vi "Dashboard Main.vi"() -> ()   [LabVIEW 2020]
uses:
  <vilib>/Utility/miscctls.llb/LVRowAndColumnTypeDef.ctl
  <vilib>/event_ctls.llb/eventvkey.ctl
  <vilib>/Rock Robotics/Network Tables/NT Read Numeric Array.vi
  AUtonomo/Robot Global Data.vi
  <vilib>/Rock Robotics/WPI/Dashboard/WPI_DashboardLogging Global.vi
panel:
  in  "Camera Settings Right":T1={"Frame Rate"=30, "Compression"=30, "Size"=1, "DB Camera Config"=FALSE} {"Frame Rate" scale=1.0..30.0; "Compression" scale=100.0..-1.0; "Size" items=["640x480", "320x240", "160x120"]}
  in  "Camera Name Right":string(combo)="No Camera Selection"
  out "Camera Perf":string
  in  "Camera Settings":T1={"Frame Rate"=30, "Compression"=30, "Size"=1, "DB Camera Config"=FALSE} {"Frame Rate" scale=1.0..30.0; "Compression" scale=100.0..-1.0; "Size" items=["640x480", "320x240", "160x120"]}
  in  "TCP":refnum<k5>
  in  "Rec Mode":enum32{"Stop", "Record", "Playback"}(radio)
  out "Robot IP":string
  out "Image Message":string="Timeout in Camera Communications"
  in  "Dashboard Tab":T2(tab)
  in  "Select Auto":string(combo)="Select Autonomous ..."
  out "NT Connection":bool
  out "MotorChart R":cluster{"Numeric":dbl, "Numeric":dbl}(graph)
  out "MotorChart L":cluster{"Numeric":dbl, "Numeric":dbl}(graph)
  out "MotorSliders R":cluster{"MotorSlide1":dbl, "MotorSlide2":dbl} {"MotorSlide2" scale=-1.0..1.0 scale format="%#_2e"; "MotorSlide1" scale=-1.0..1.0 scale format="%#_2e"}
  out "MotorSliders L":cluster{"MotorSlide1":dbl, "MotorSlide2":dbl} {"MotorSlide2" scale=-1.0..1.0 scale format="%#_2e"; "MotorSlide1" scale=-1.0..1.0 scale format="%#_2e"}
  out "Gyro":dbl(knob) scale=0.0..360.0
  out "JS1 Z":dbl(slide) scale=-1.0..1.0 scale format="%#_2e"
  out "JS1 Graph":cluster{"X":dbl, "Y":dbl}[](graph)
  out "JS1 Buttons":T3
  out "JS2 Z":dbl(slide) scale=-1.0..1.0 scale format="%#_2e"
  out "JS2 Graph":cluster{"X":dbl, "Y":dbl}[](graph)
  out "JS2 Buttons":T3
  out "Mode":T4(ring)=enum."Auto Disabled"
  out "Right Camera Perf":cluster{"Bandwidth (Mbps)":dbl, "FPS":dbl}
  out "Camera Image Right":T5(plugin-control)
  in  "DB/String 9":string
  in  "DB/String 8":string
  in  "DB/String 7":string
  in  "DB/String 6":string
  in  "DB/String 5":string
  in  "DB/String 4":string
  in  "DB/String 3":string
  in  "DB/String 2":string
  in  "DB/String 1":string
  in  "DB/String 0":string
  in  "DB/Slider 0":dbl(slide) scale=0.0..5.0
  in  "DB/Slider 1":dbl(slide) scale=0.0..5.0
  in  "DB/Slider 2":dbl(slide) scale=0.0..5.0
  in  "DB/Slider 3":dbl(slide) scale=0.0..5.0
  out "DB/LED 3":bool
  out "DB/LED 2":bool
  out "DB/LED 1":bool
  out "DB/LED 0":bool
  in  "DB/Button 3":bool
  in  "DB/Button 2":bool
  in  "DB/Button 1":bool
  in  "DB/Button 0":bool caption="New Name"
  in  "Test Slider":dbl(slide) scale=0.0..100.0 scale format="%#_3g"
  in  "On/Off":bool caption="Solenoid"
  in  "Test Name":u16(ring) items=["Select the test to run..."]
  in  "Test Tree":string(tree)
  in  "Motor":cluster{"Value":dbl, "Enable":bool} {"Value" scale=-1.0..1.0 scale format="%#_3g"}
  out "Progress":T6 {"Test Progress" scale=0.0..100.0}
  in  "Rev/Fwd":cluster{"Forward":bool, "Reverse":bool}
  in  "Test Ring":u16(ring) items=["Monochrome", "Color"]
  out "Cmd Status":string
  in  "Execute Command":bool
  in  "Command Params":string[][](table)
  in  "Command Selection":i32(listbox)
  in  "CheckList":i32(listbox)
  out "Tree":string(tree)
  out "Camera Image":T5(plugin-control)
  out "Background":bool
  in  "Camera Name":string(combo)="No Camera Selection"
  # "HW"
  # "HW"
  # "Joysticks"
  # "Drive Motors"
  # "Front"
  # "Right"
  # "Left"
  # "Back"
  # "This tab is a great place for autonomous settings and robot-specific values.\nPlace controls and indicators inside this tab and match name to\nDashboard Variables on robot. You can also delete this comment."
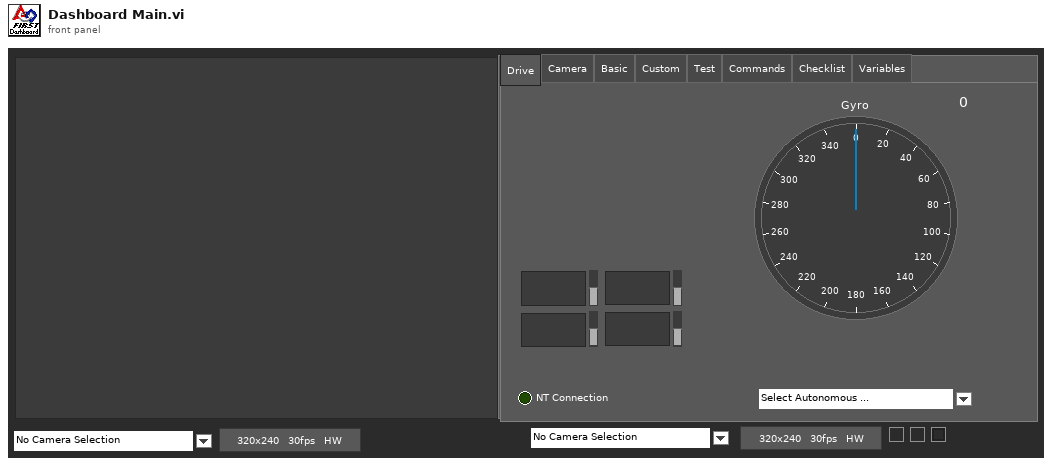
[diagram p1: front panel]
types:
  T1 = cluster{"Frame Rate":i32, "Compression":i32, "Size":u16, "DB Camera Config":bool}
  T2 = enum32{"Drive", "Camera", "Basic", "Custom", "Test", "Commands", "Checklist", "Variables"}
  T3 = cluster{bool, bool, bool, bool, bool, bool, bool, bool, bool, bool, bool, bool}
  T4 = enum8{"Tele-Op Disabled", "Tele-Op Enabled", "Auto Disabled", "Auto Enabled", "Test Disabled", "Test Enabled", "Disconnected", "No Code", "E-Stop"}
  T5 = typedef "IMAQ Image.ctl" = refnum<image>
  T6 = cluster{"Test Progress":u8, "Test Progress Text":string}
  T7 = cluster{"Save Path":path, "Interval (s)":dbl, "Keep":i32}
  T8 = typedef "Image Type" = u32
  T9 = cluster{"IDs":cluster{"RPC field ID":u16, "Unique ID":u16}, "String":string}
  T10 = cluster{"Error Strings":string, "Disable Counts":cluster{u16, u16}, "Rail Faults":cluster{u16, u16, u16}, "Robot IP":string, "DB Mode":u8, "Event Info":cluster{"Name":string, "Type":u8, "Number":u16, "Replay":u8}}
  T11 = cluster{"Storage":cluster{"Disk Free":u64, "RAM Block":u32, "RAM free":u32}, "CPU Utilization":cluster{"CPU % ISR":sgl, "CPU % Time Crit":sgl, "CPU % Timed Str":sgl, "CPU % High":sgl, "CPU % Above":sgl, "CPU % Normal":sgl, "CPU % Low":sgl}, "CAN":cluster{"% Bus Utilization":sgl, "Bus Off Cnt":u32, "TX_FIFO Full Cnt":u32, "Receive Error Cnt":u8, "Transmit Error Cnt":u8}, "HID":cluster{"HID Outputs":u32, "Rumble Low":u16, "Rumble High":u16}[]}
  T12 = cluster{"Status bits":cluster{"Test Mode":bool, "Autonomous":bool, "Enabled":bool, "Code Start":bool, "Brownout":bool, "Reserved 2":bool, "Reserved 3":bool, "E-Stop":bool}, "Code Trace":cluster{"Disabled":bool, "TeleOp":bool, "Auto":bool, "Test":bool}, "Controller Type":enum16{"unknown", "cRIO", "roboRio"}, "Code?":enum16{"unknown", "noCode", "code"}, "Battery V":dbl}
  T13 = cluster{"Control Bits":cluster{"TestMode":bool, "Autonomous":bool, "Enabled":bool, "FMS Present":bool, bool, bool, bool, "E-Stop":bool}, "Team Station ":u8, "Countdown":sgl, "Joystick Values":cluster{"Axes":dbl[], "Buttons":bool[], "POVs":i16[]}[]}
  T14 = cluster{"Axes":dbl[], "Buttons":bool[], "POVs":i16[]}[]
  T15 = cluster{"Axes":dbl[], "Buttons":bool[], "POVs":i16[]}
  T16 = cluster{"Buttons[0]":bool, "Buttons[1]":bool, "Buttons[2]":bool, "Buttons[3]":bool, "Buttons[4]":bool, "Buttons[5]":bool, "Buttons[6]":bool, "Buttons[7]":bool, "Buttons[8]":bool, "Buttons[9]":bool, "Buttons[10]":bool, "Buttons[11]":bool}
  T17 = cluster{"Camera Image":refnum<vi>, "Dashboard Tab":refnum<vi>, "Background":refnum<vi>, "Rec Mode":refnum<vi>, "Test Slider":refnum<vi>, "On/Off ":refnum<vi>, "Test Ring":refnum<vi>, "Rev/Fwd":refnum<vi>, "Test Name":refnum<vi>, "Motor":refnum<vi>, "Progress":refnum<vi>, "CheckList":refnum<vi>, "Tree":refnum<vi>, "Test Tree":refnum<vi>, "Command Params":refnum<vi>, "Command Selection":refnum<vi>, "Execute Command":refnum<vi>, "Cmd Status":refnum<vi>, "Camera Settings":refnum<vi>, "Camera Name":refnum<vi>, "Camera Perf":refnum<vi>, "Camera Settings Right":refnum<vi>, "Camera Name Right":refnum<vi>, "Camera Image Right":refnum<vi>}
  T18 = cluster{"Global Rectangle":i32[], "Contours":cluster{"Contour Type":u32, "ROI Type":u32, "Points":i32[]}[]}
  T19 = cluster{"Camera Name":string, string, "Saved DB Images Info":cluster{"Save Path":path, "Interval (s)":dbl, "Keep":i32}}
  T20 = cluster{"Camera Name Right":string, string, "Saved DB Images Info":cluster{"Save Path":path, "Interval (s)":dbl, "Keep":i32}}
  T21 = cluster{"Operation":enum16{"Update", "Clear"}, "Color Box":u32}[]
  T22 = typedef "eventvkey.ctl" = enum16{"ASCII", "Enter", "Return", "Shift", "Ctrl", "Alt", "Cmd", "Opt", "Caps", "NumLock", "Clear", "Break", "Up", "Down", "Left", "Right", "Insert", "Delete", "Home", "End", "PageUp", "PageDown", "Escape", "Help", "Pause", "ScrollLock", "F1", "F2", "F3", "F4", "F5", "F6", "F7", "F8", "F9", "F10", "F11", "F12", "F13", "F14", "F15", "F16", "F17", "F18", "F19", "F20", "F21", "F22", "F23", "F24", "Play", "VolumeUp", "VolumeDown", "Mute", "Two Byte Char"}
  T23 = cluster{"Image Size":bool, "Image Type":bool, "Pixel Value":bool, "ROI Information":bool, "Zoom Factor":bool}
  T24 = cluster{"Operation":enum16{"Update", "Clear"}, "Color Box":u32}
  T25 = typedef "LVRowAndColumnTypeDef.ctl" = cluster{"Row":i32, "Column":i32}
  T26 = cluster{"Shift":bool, "Ctrl":bool, "Alt":bool, "Cmd":bool, "Opt":bool}
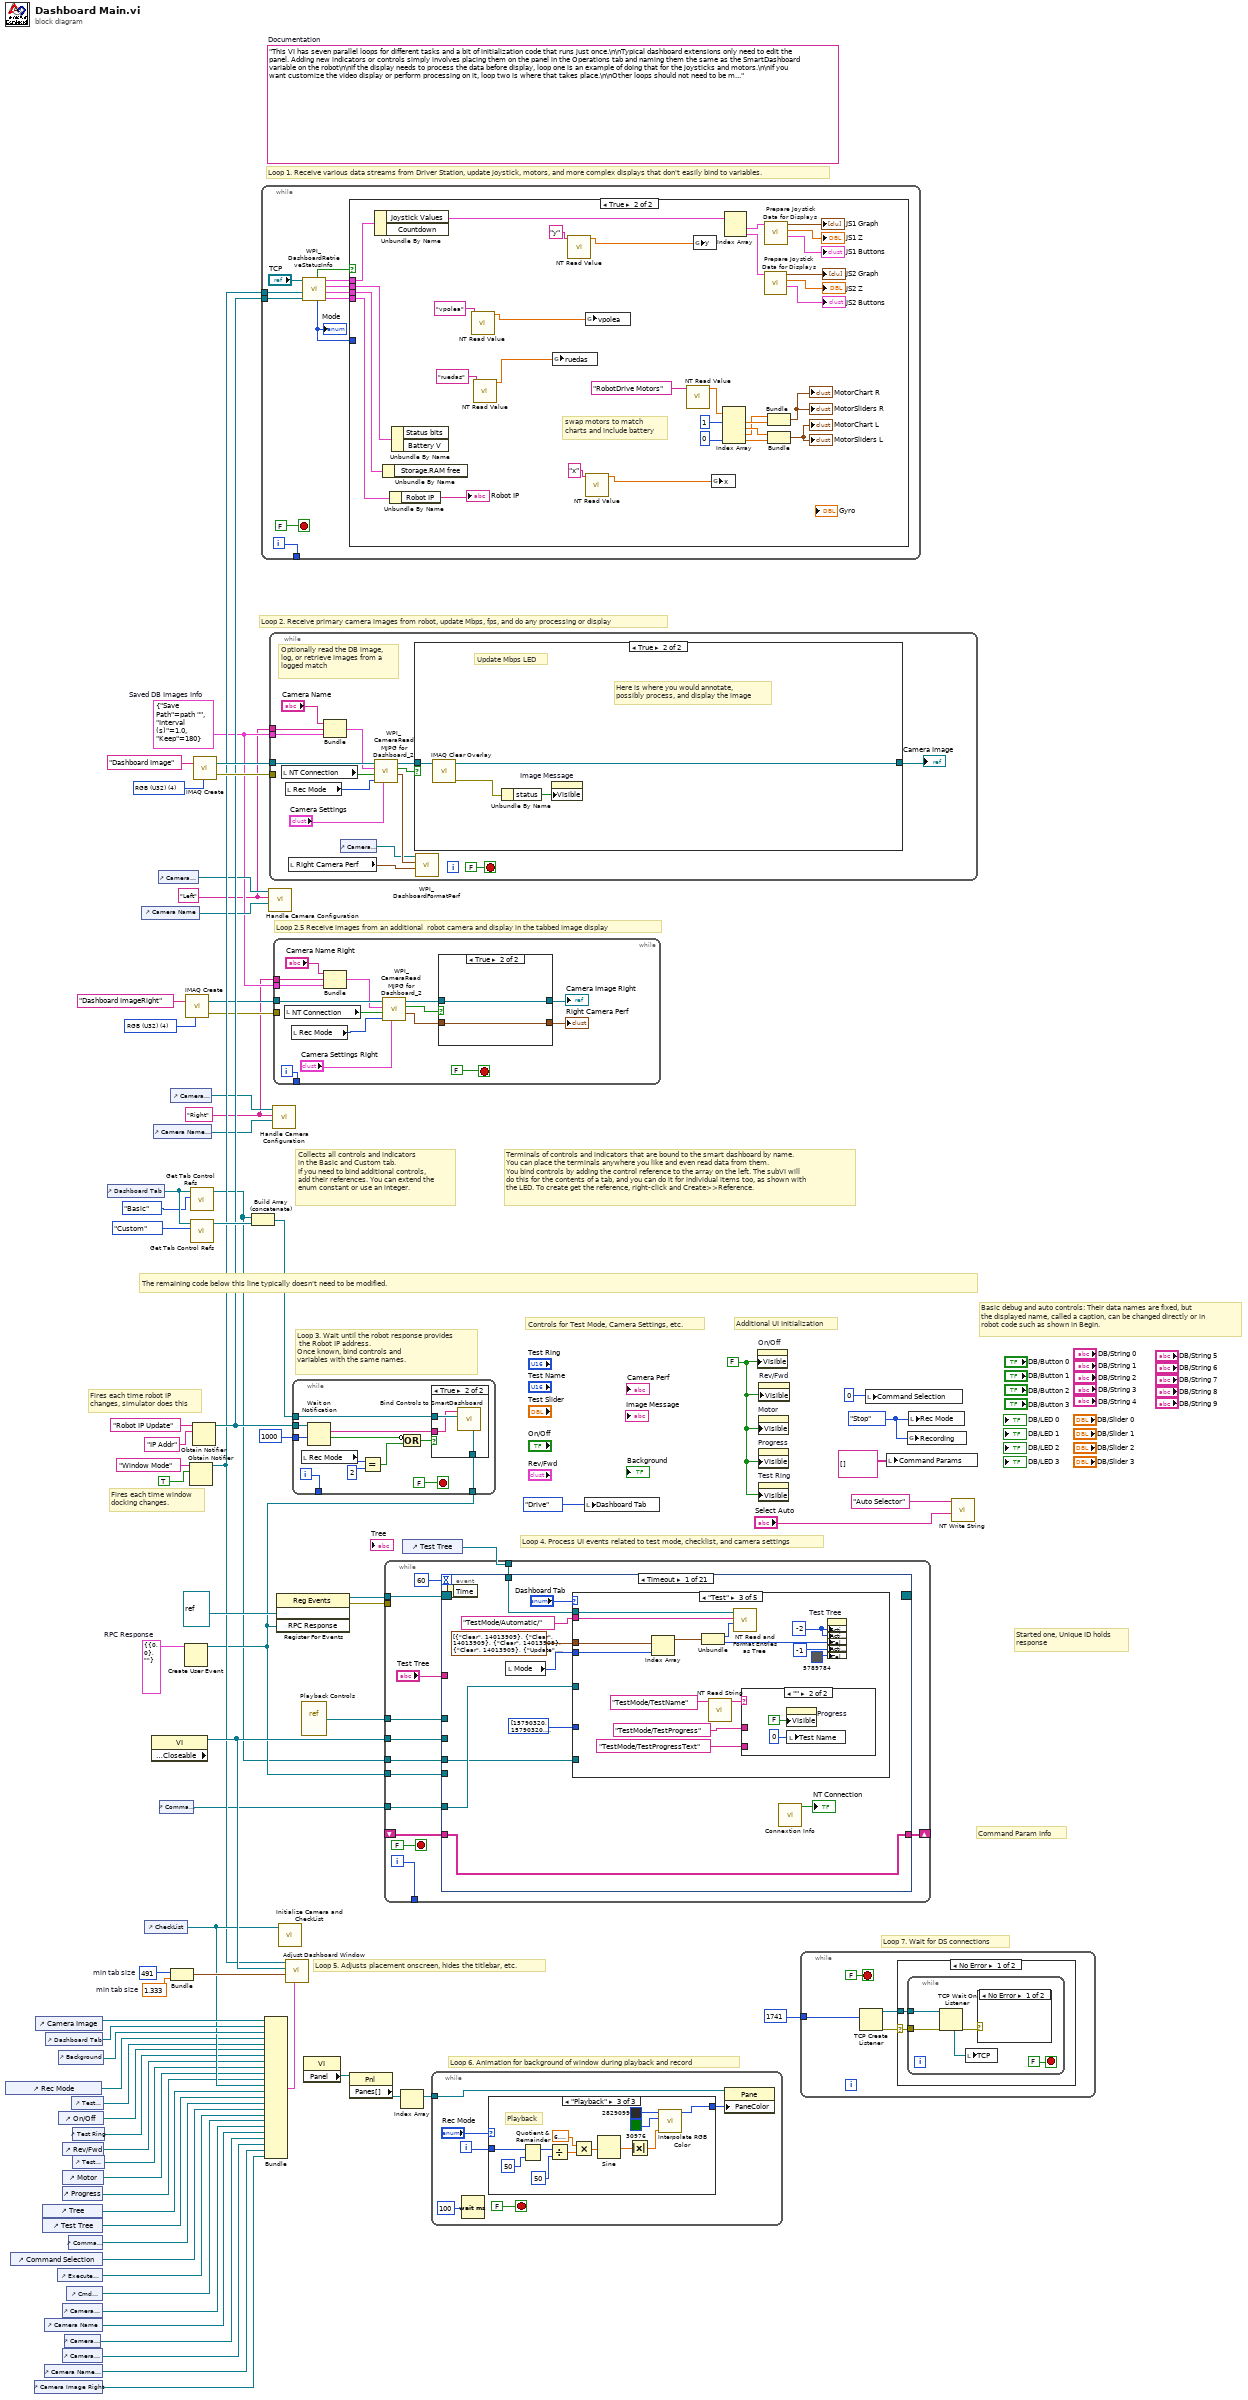
[diagram p0: block diagram]
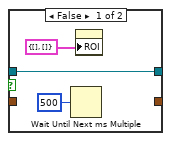
[diagram p2: hidden frame]
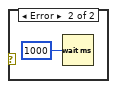
[diagram p3: hidden frame]
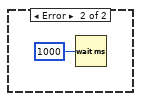
[diagram p4: hidden frame]
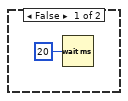
[diagram p5: hidden frame]
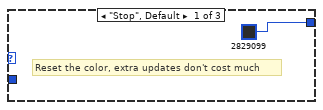
[diagram p6: hidden frame]
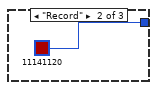
[diagram p7: hidden frame]
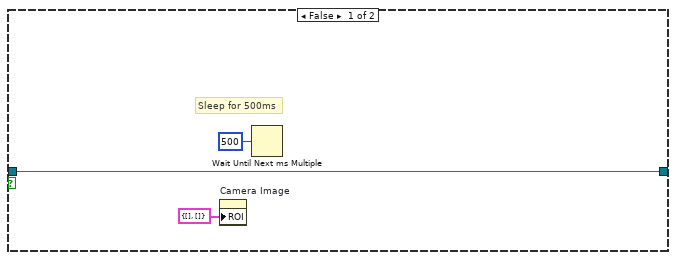
[diagram p9: hidden frame]
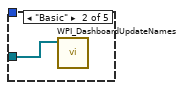
[diagram p11: hidden frame]
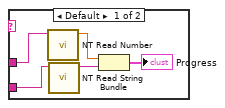
[diagram p12: hidden frame]
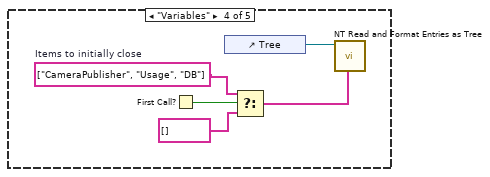
[diagram p13: hidden frame]
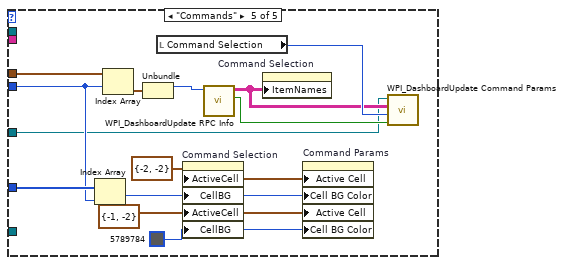
[diagram p14: hidden frame]
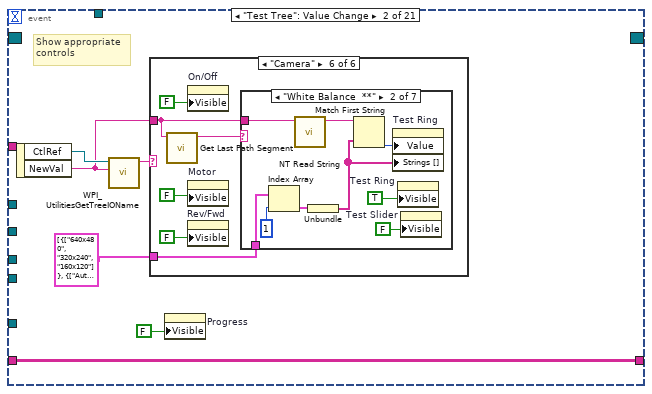
[diagram p15: hidden frame]
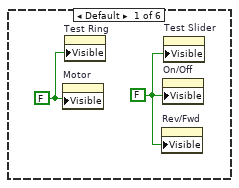
[diagram p16: hidden frame]
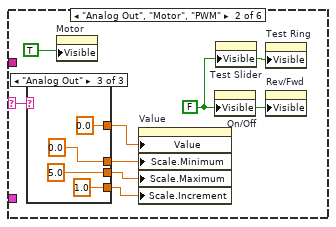
[diagram p17: hidden frame]
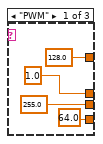
[diagram p18: hidden frame]
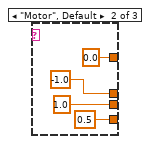
[diagram p19: hidden frame]
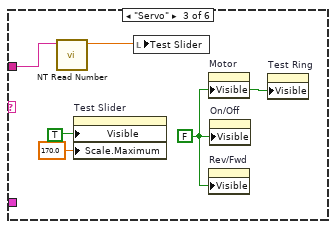
[diagram p20: hidden frame]
diagram:
  w3 = T7 {"Save Path"=path "", "Interval (s)"=1.0, "Keep"=180}  # Saved DB Images Info
  w2 = "Right"
  w1 = "Left"
  w13 = T8 4 items=["Grayscale (U8)", "Grayscale (I16)", "Grayscale (SGL)", "Complex (CSG)", "RGB (U32)", "HSL (U32)", "RGB (U64)"] ("Image Type")
  w29 = T9 {"IDs"={"RPC field ID"=0, "Unique ID"=0}, "String"=""}  # RPC Response
  w52 = 491  # min tab size
  w51 = 1.333  # min tab size
  w59 = enum32{"Stop", "Record", "Playback"}."Stop" ("Rec Mode")
  w36 = FALSE ("Visible")
  (unwired) "This VI has seven parallel loops for different tasks and a bit of initialization code that runs just once.\n\nTypical dashboard extensions only need to edit the panel. Adding new indicators or controls simply involves placing them on the panel in the Operations tab and naming them the same as the SmartDashboard variable on the robot\n\nIf the display needs to process the data before display, loop one is an example of doing that for the joysticks and motors.\n\nIf you want customize the video display or perform processing on it, loop two is where that takes place.\n\nOther loops should not need to be modified. They are pretty standard, and document the task they perform."  # Documentation
  w76 = T8 4 items=["Grayscale (U8)", "Grayscale (I16)", "Grayscale (SGL)", "Complex (CSG)", "RGB (U32)", "HSL (U32)", "RGB (U64)"] ("Image Type")
  # "Loop 2.5 Receive images from an additional  robot camera and display in the tabbed image display"
  # "Command Param Info"
  # "Started one, Unique ID holds\nresponse"
  # "Loop 7. Wait for DS connections"
  # "Basic debug and auto controls: Their data names are fixed, but\nthe displayed name, called a caption, can be changed directly or in\nrobot code such as shown in Begin."
  # "Controls for Test Mode, Camera Settings, etc."
  # "Additional UI Initialization"
  # "Loop 6. Animation for background of window during playback and record"
  # "Fires each time robot IP\nchanges, simulator does this"
  # "Fires each time window\ndocking changes."
  # "Collects all controls and indicators\nin the Basic and Custom tab.\nIf you need to bind additional controls,\nadd their references. You can extend the\nenum constant or use an integer."
  # "The remaining code below this line typically doesn't need to be modified."
  # "Loop 4. Process UI events related to test mode, checklist, and camera settings"
  # "Terminals of controls and indicators that are bound to the smart dashboard by name.\nYou can place the terminals anywhere you like and even read data from them.\nYou bind controls by adding the control reference to the array on the left. The subVI will\ndo this for the contents of a tab, and you can do it for individual items too, as shown with\nthe LED. To create get the reference, right-click and Create>>Reference."
  # "Loop 3. Wait until the robot response provides\n the Robot IP address.\nOnce known, bind controls and\nvariables with the same names."
  # "Loop 5. Adjusts placement onscreen, hides the titlebar, etc."
  # "Loop 1. Receive various data streams from Driver Station, update joystick, motors, and more complex displays that don't easily bind to variables."
  # "Loop 2. Receive primary camera images from robot, update Mbps, fps, and do any processing or display"
  n1 = control-ref of="Rec Mode"() -> (w42:refnum<vi>)
  n2 = control-ref of="Command Selection"() -> (w28:refnum<vi>)
  n3 = control-ref of="Camera Image Right"() -> (w6:refnum<vi>)
  n4 = control-ref of="Camera Image"() -> (w54:refnum<vi>)
  n5 = control-ref of="Tree"() -> (w46:refnum<vi>)
  n6 = control-ref of="Test Tree"() -> (w45:refnum<vi>)
  n7 = control-ref of="Camera Name"() -> (w19:refnum<vi>)
  n8 = control-ref of="Camera Name Right"() -> (w7:refnum<vi>)
  n9 = control-ref of="Dashboard Tab"() -> (w53:refnum<vi>)
  n10 = control-ref of="Execute Command"() -> (w30:refnum<vi>)
  n11 = control-ref of="Background"() -> (w49:refnum<vi>)
  n12 = control-ref of="On/Off"() -> (w40:refnum<vi>)
  n13 = control-ref of="Progress"() -> (w37:refnum<vi>)
  n14 = control-ref of="Camera Settings"() -> (w20:refnum<vi>)
  n15 = control-ref of="Camera Settings Right"() -> (w8:refnum<vi>)
  n16 = control-ref of="Rev/Fwd"() -> (w38:refnum<vi>)
  n17 = control-ref of="Motor"() -> (w43:refnum<vi>)
  n18 = control-ref of="Camera Perf"() -> (w18:refnum<vi>)
  n19 = control-ref of="Cmd Status"() -> (w24:refnum<vi>)
  n20 = control-ref of="Command Params"() -> (w31:refnum<vi>)
  n21 = control-ref of="Test Slider"() -> (w41:refnum<vi>)
  n22 = control-ref of="Test Ring"() -> (w39:refnum<vi>)
  n23 = control-ref of="Test Name"() -> (w44:refnum<vi>)
  n24 = control-ref of="Dashboard Tab"() -> (w57:refnum<vi>)
  n25 = control-ref of="Camera Name"() -> (w21:refnum<vi>)
  n26 = control-ref of="CheckList"() -> (w47:refnum<vi>)
  n27 = property class="VI" props=["Front Panel.Closeable"]() -> (reference out=w58:refnum<vi>)  [unwired: 2 in, 2 out]
  n28 = control-ref of="Camera Name Right"() -> (w9:refnum<vi>)
  n29 = control-ref of="Camera Settings"() -> (w22:refnum<vi>)
  n30 = control-ref of="Command Params"() -> (w23:refnum<vi>)
  n31 = control-ref of="Camera Settings Right"() -> (w10:refnum<vi>)
  n32 = Bundle("min tab size"=w52, "min tab size"=w51) -> (w50:cluster{"min tab size":i32, "min tab size":dbl})  [unwired: 1 in]
  n33 = Create User Event(user event datatype=w29) -> (user event=w25:refnum<user-event>)  [unwired: 1 in, 1 out]
  n34 = call "IMAQ Create"("Image Name"="Dashboard ImageRight", "Image Type"=w13) -> ("New Image"=w12:T5, "error out"=w11:errorcluster)  [unwired: 2 in, 1 out]
  n35 = Obtain Notifier(name (unnamed)="Window Mode", notification data type=TRUE) -> (notifier out=w34:refnum<notifier>)  [unwired: 2 in, 2 out]
  n36 = call <vilib>:"Get Tab Control Refs.vi"("Page Index"=T2."Basic" ("Dashboard Tab"), "TabControl in"=w57) -> ("ControlsOnPage"=w17:refnum<vi>[])  [unwired: 9 in]
  n37 = call <vilib>:"Get Tab Control Refs.vi"("Page Index"=T2."Custom" ("Dashboard Tab"), "TabControl in"=w57) -> ("ControlsOnPage"=w56:refnum<vi>[])  [unwired: 9 in]
  n38 = Obtain Notifier(name (unnamed)="Robot IP Update", notification data type="IP Addr" ("name (unnamed)")) -> (notifier out=w35:refnum<notifier>)  [unwired: 2 in, 2 out]
  n39 = call "IMAQ Create"("Image Name"="Dashboard Image", "Image Type"=w76) -> ("New Image"=w74:T5, "error out"=w73:errorcluster)  [unwired: 2 in, 1 out]
  n40 = Build Array (concatenate)(w17, w56) -> (w55:refnum<vi>[])
  n41 = while {
    tunnel: [w86] -> _
    tunnel: w35 -> [w80]
    tunnel: w34 -> [w77]
    i -> [w86]
    stop <- FALSE stop-if-true
    n42 = call <vilib>:"WPI_DashboardRetrieveStatusInfo.vi"("Binding Refnum"=w80, "Window Mode Notifier"=w77, "TCP Cnx"="TCP") -> ("Power and Errors"=w81:T10, "Robot Metrics"=w84:T11, "Status Info"=w85:T12, "Control Info"=w82:T13, "Robot Mode"=w79:T4, "Process?"=w83:bool)  [unwired: 3 in]
    "Mode" <- w79
    n43 = case shown="True" w83 {
      tunnel: w85 -> [_ w120]
      tunnel: w84 -> [_ w119]
      tunnel: w82 -> [_ w118]
      tunnel: w81 -> [_ w117]
      tunnel: w79 -> [_ _]
      frame False {
        n44 = Wait (ms)(milliseconds to wait=u32 20) -> ()  [unwired: 1 out]
      }
      frame True {
        # "swap motors to match\ncharts and include battery"
        n45 = Unbundle By Name(w118) -> ("Joystick Values"=w108:T14)  [unwired: 1 out]
        n46 = Unbundle By Name(w119) -> ()  [unwired: 1 out]
        n47 = Unbundle By Name(w117) -> ("Robot IP"=→"Robot IP":string)
        n48 = Unbundle By Name(w120) -> ()  [unwired: 2 out]
        n49 = call-poly <vilib>:"NT Read Value.vi"("Name"="vpolea") -> ("Numeric"=w94:dbl)  [unwired: 9 in, 1 out]
        n50 = call-poly <vilib>:"NT Read Value.vi"("Name"="ruedas") -> ("Numeric"=w93:dbl)  [unwired: 9 in, 1 out]
        n51 = global write "Robot Global Data.vi" "ruedas"(w93) -> ()
        n52 = call-poly <vilib>:"NT Read Value.vi"("Name"="y") -> ("Numeric"=w90:dbl)  [unwired: 9 in, 1 out]
        n53 = global write "Robot Global Data.vi" "vpolea"(w94) -> ()
        n54 = call-poly <vilib>:"NT Read Value.vi"("Name"="x") -> ("Numeric"=w92:dbl)  [unwired: 9 in, 1 out]
        n55 = call-poly <vilib>:"NT Read Value.vi"("Name"="RobotDrive Motors") -> ("Numeric Array"=w98:dbl[])  [unwired: 9 in, 1 out]
        n56 = global write "Robot Global Data.vi" "y"(w90) -> ()
        n57 = global write "Robot Global Data.vi" "x"(w92) -> ()
        n58 = Index Array(array=w98, index #1=1, index #4=0) -> (element #1=w112:dbl, element #2=w113:dbl, element #3=w111:dbl, element #4=w116:dbl)  [unwired: 2 in]
        n59 = Index Array(array=w108) -> (element #1=w107:T15, element #2=w103:T15)  [unwired: 2 in]
        n60 = call "Prepare Joystick Data for Displays.vi"("Joystick Values"=w103) -> ("Buttons"=→"JS2 Buttons":T16, "Z Axis"=→"JS2 Z":dbl, "Cartesian Data"=→"JS2 Graph":cluster{"X axis":dbl, "X axis":dbl}[])  [unwired: 8 in]
        n61 = call "Prepare Joystick Data for Displays.vi"("Joystick Values"=w107) -> ("Buttons"=→"JS1 Buttons":T16, "Z Axis"=→"JS1 Z":dbl, "Cartesian Data"=→"JS1 Graph":cluster{"X axis":dbl, "X axis":dbl}[])  [unwired: 8 in]
        n62 = Bundle("Numeric"=w111, "Numeric"=w112) -> (→"MotorChart R" →"MotorSliders R":cluster{"Numeric":dbl, "Numeric":dbl})  [unwired: 1 in]
        n63 = Bundle("Numeric"=w113, "Numeric"=w116) -> (→"MotorChart L" →"MotorSliders L":cluster{"Numeric":dbl, "Numeric":dbl})  [unwired: 1 in]
      }
    }
  }
  n64 = Bundle("Camera Image"=w54, "Dashboard Tab"=w53, "Background"=w49, "Rec Mode"=w42, "Test Slider"=w41, "On/Off"=w40, "Test Ring"=w39, "Rev/Fwd"=w38, "Test Name"=w44, "Motor"=w43, "Progress"=w37, "CheckList"=w47, "Tree"=w46, "Test Tree"=w45, "Command Params"=w31, "Command Selection"=w28, "Execute Command"=w30, "Cmd Status"=w24, "Camera Settings"=w20, "Camera Name"=w19, "Camera Perf"=w18, "Camera Settings Right"=w8, "Camera Name Right"=w7, "Camera Image Right"=w6) -> (w48:T17)  [unwired: 1 in]
  n65 = call "Handle Camera Configuration.vi"("CameraNameRef"=w21, "Display Name"=w1, "ClusterRef"=w22) -> ()  [unwired: 9 in]
  n66 = while {
    tunnel: w74 -> [w134]
    tunnel: w73 -> [_]
    tunnel: w3 -> [w127]
    tunnel: w1 -> [w124]
    stop <- FALSE stop-if-true
    # "Optionally read the DB image,\nlog, or retrieve images from a\nlogged match"
    n67 = local read "NT Connection"() -> (w128:bool)
    n68 = local read "Rec Mode"() -> (w131:enum32{"Stop", "Record", "Playback"})
    n69 = local read "Right Camera Perf"() -> (w122:cluster{"Bandwidth (Mbps)":dbl, "FPS":dbl})
    n70 = Bundle("Camera Name"="Camera Name", w124, "Saved DB Images Info"=w127) -> (w126:T19)  [unwired: 1 in]
    n71 = control-ref of="Camera Perf"() -> (w121:refnum<vi>)
    n72 = call <vilib>:"WPI_CameraRead MJPG for Dashboard_2.vi"("Camera Settings"="Camera Settings", "Rec Mode"=w131, "NT Connection"=w128, "Capture Info"=w126, "Image in"=w134) -> ("perf info"=w123:cluster{"Bandwidth (Mbps)":dbl, "fps":dbl}, "Active"=w132:bool, "Image\\ out"=w133:T5)  [unwired: 4 in]
    n73 = case shown="True" w132 {
      tunnel: w133 -> [w137 w140]
      tunnel: [w137 w139] -> w129
      frame False {
        # "Sleep for 500ms"
        n74 = property on="Camera Image" class="ImageControl"("ROI"=T18 {"Global Rectangle"=[], "Contours"=[]}) -> ()  [unwired: 2 in, 2 out]
        n75 = Wait Until Next ms Multiple(millisecond multiple=u32 500) -> ()  [unwired: 1 out]
      }
      frame True {
        # "Here is where you would annotate,\npossibly process, and display the image"
        # "Update Mbps LED"
        n76 = call "IMAQ Clear Overlay"("Image"=w140) -> ("error out"=w141:errorcluster, "Image Out"=w139:T5)  [unwired: 2 in, 7 out]
        n77 = Unbundle By Name(w141) -> ("status"=w142:bool)
        n78 = property on="Image Message" class="Str"("Visible"=w142) -> ()  [unwired: 2 in, 2 out]
      }
    }
    "Camera Image" <- w129
    n79 = call <vilib>:"WPI_DashboardFormatPerf.vi"("Right Camera Perf"=w122, "Performance"=w123, "String in"=w121) -> ()  [unwired: 9 in]
  }
  n80 = call "Handle Camera Configuration.vi"("CameraNameRef"=w9, "Display Name"=w2, "ClusterRef"=w10) -> ()  [unwired: 9 in]
  n81 = while {
    tunnel: w12 -> [w157]
    tunnel: w11 -> [_]
    tunnel: [w152] -> _
    tunnel: w3 -> [w148]
    tunnel: w2 -> [w145]
    i -> [w152]
    stop <- FALSE stop-if-true
    n82 = local read "NT Connection"() -> (w149:bool)
    n83 = local read "Rec Mode"() -> (w156:enum32{"Stop", "Record", "Playback"})
    n84 = Bundle("Camera Name Right"="Camera Name Right", w145, "Saved DB Images Info"=w148) -> (w147:T20)  [unwired: 1 in]
    n85 = call <vilib>:"WPI_CameraRead MJPG for Dashboard_2.vi"("Camera Settings"="Camera Settings Right", "Rec Mode"=w156, "NT Connection"=w149, "Capture Info"=w147, "Image in"=w157) -> ("perf info"=w143:cluster{"Bandwidth (Mbps)":dbl, "fps":dbl}, "Active"=w151:bool, "Image\\ out"=w154:T5)  [unwired: 4 in]
    n86 = case shown="True" w151 {
      tunnel: w154 -> [w159 w162]
      tunnel: [w159 w162] -> w150
      tunnel: [_ w161] -> w144
      tunnel: w143 -> [_ w161]
      frame False {
        n87 = Wait Until Next ms Multiple(millisecond multiple=u32 500) -> ()  [unwired: 1 out]
        n88 = property on="Camera Image Right" class="ImageControl"("ROI"=T18 {"Global Rectangle"=[], "Contours"=[]}) -> ()  [unwired: 2 in, 2 out]
      }
      frame True {
      }
    }
    "Camera Image Right" <- w150
    "Right Camera Perf" <- w144
  }
  n89 = register-events(refnum<vi> refnum, w25) -> (reference out=w63:refnum<event-registration>, error out=w62:errorcluster)  [unwired: 2 in]
  n90 = call "Initialize Camera and CheckList.vi"("ListBox in"=w47) -> ()  [unwired: 11 in]
  n91 = call "Adjust Dashboard Window.vi"("Sizing Refnums"=w48, "Size Constraints"=w50, "VI"=w58, "WIn Mode"=w34) -> ()  [unwired: 8 in]
  n92 = while {
    tunnel: w55 -> [w174]
    tunnel: w35 -> [w172]
    tunnel: [w170] -> _
    tunnel: u32 1000 ("milliseconds to wait") -> [w169]
    tunnel: w25 -> [w163]
    i -> [w170]
    stop <- FALSE stop-if-true
    n93 = local read "Rec Mode"() -> (w165:enum32{"Stop", "Record", "Playback"})
    n94 = Wait on Notification(notifier=w172, timeout in ms (-1)=w169) -> (notification=w171:string, timed out?=w167:bool)  [unwired: 2 in, 2 out]
    n95 = Equal?(x=w165, y=u16 2 ("Rec Mode")) -> (x = y?=w166:bool)
    n96 = Compound Arithmetic op=OR(invert w167, w166) -> (w168:bool)
    n97 = case shown="True" w168 {
      tunnel: w174 -> [_ w177]
      tunnel: w171 -> [_ w176]
      tunnel: w163 -> [_ w175]
      frame False {
      }
      frame True {
        n98 = call <vilib>:"Bind Controls to SmartDashboard.vi"("RPC ref"=w175, "Bound Control Refs"=w177, "Server IP Address"=w176) -> ()  [unwired: 9 in]
      }
    }
  }
  n99 = vi-ref "Playback Controls.vi"() -> (w64:refnum<vi>)
  n100 = property class="VI"() -> ("Panel"=w66:refnum<vi>)  [unwired: 2 in, 2 out]
  n101 = property class="Pnl"(reference=w66) -> ("Panes[]"=w67:refnum<vi>[])  [unwired: 1 in, 2 out]
  n102 = Index Array(array=w67) -> (element=w65:refnum<vi>)  [unwired: 1 in]
  n103 = control-ref of="Test Tree"() -> (w68:refnum<vi>)
  n104 = while {
    tunnel: [w187] -> _
    tunnel: w68 -> [w186]
    tunnel: w64 -> [w185]
    tunnel: w63 -> [w184]
    tunnel: w62 -> [_]
    tunnel: w58 -> [w183]
    tunnel: w25 -> [w182]
    tunnel: w23 -> [w181]
    shift-right: [w180] -> _
    shift-left: _ -> [w179]
    tunnel: w17 -> [w178]
    i -> [w187]
    stop <- FALSE stop-if-true
    n105 = event shown="[0] Timeout" {
      selector: w184 -> [_ _ _ _ _ _ _ _ _ _ _ _ _ _ _ _ _ _ _ _ _]
      dyn-events: [_ _ _ _ _ _ _ _ _ _ _ _ _ _ _ _ w447 _ _ _ _] -> _
      timeout: u32 60 ("milliseconds to wait") -> [_ _ _ _ _ _ _ _ _ _ _ _ _ _ _ _ _ _ _ _ _]
      tunnel: w186 -> [w199 _ _ _ _ _ _ _ _ _ _ _ _ _ _ _ _ _ _ _ _]
      tunnel: "Test Tree" -> [_ _ _ _ _ _ _ _ _ _ _ w414 w422 w424 w428 w436 _ _ _ _ _]
      tunnel: w185 -> [_ _ _ _ _ _ _ _ _ _ _ _ _ _ _ _ w449 _ w467 _ _]
      tunnel: w183 -> [_ _ _ _ _ _ _ _ _ _ _ _ _ _ _ _ w445 _ _ _ _]
      tunnel: w182 -> [_ _ _ _ _ _ _ _ _ _ _ _ _ _ _ _ w443 _ _ _ _]
      tunnel: w181 -> [w194 _ _ _ _ _ w365 _ _ _ _ _ _ _ _ _ _ _ _ _ _]
      tunnel: [w193 w242 w344 w349 w358 w362 w363 w372 w382 w389 w401 w413 w420 w423 w427 w435 w442 w462 w464 w468 w481] -> w180
      tunnel: w179 -> [w193 w242 w344 w349 w358 w362 w363 _ _ w389 w401 w413 w420 w423 w427 w435 w442 w462 w464 w468 w481]
      tunnel: w178 -> [w191 _ _ _ _ _ _ _ _ _ _ _ _ _ _ _ _ _ _ _ _]
      event Timeout {
        n106 = event-data() -> ()  [unwired: 1 in, 1 out]
        n107 = local read "Mode"() -> (w196:T4)
        n108 = case shown="\"Test\"" "Dashboard Tab" {
          tunnel: w199 -> [_ _ w215 _ _]
          tunnel: "TestMode/Automatic/" ("Name Pattern") -> [_ _ w214 _ _]
          tunnel: T21 [{"Operation"=enum."Clear", "Color Box"=14013909}, {"Operation"=enum."Clear", "Color Box"=14013909}, {"Operation"=enum."Clear", "Color Box"=14013909}, {"Operation"=enum."Clear", "Color Box"=14013909}, {"Operation"=enum."Update", "Color Box"=14013909}, {"Operation"=enum."Update", "Color Box"=16777215}, {"Operation"=enum."Clear", "Color Box"=14013909}, {"Operation"=enum."Clear", "Color Box"=14013909}, {"Operation"=enum."Clear", "Color Box"=14013909}] -> [_ _ w207 _ w235]
          tunnel: w196 -> [_ _ w206 _ w234]
          tunnel: u32[] [15790320, 15790320, 15790320, 15790320, 16777215, 16777215, 15790320, 15790320, 15790320] -> [_ _ _ _ w240]
          tunnel: w194 -> [_ _ _ _ w228]
          tunnel: w191 -> [_ w201 _ _ _]
          frame "Custom", Default {
          }
          frame "Basic" {
            n109 = call <vilib>:"WPI_DashboardUpdateNames.vi"("Controls on Tab"=w201) -> ()  [unwired: 11 in]
          }
          frame "Test" {
            w213 = -2 ("Active Item:Row Number")
            n110 = Index Array(array=w207, index=w206) -> (element=w208:T24)
            n111 = Unbundle(w208) -> ("Operation"=w209:enum16{"Update", "Clear"}, "Color Box"=w210:u32)
            n112 = call <vilib>:"NT Read String.vi"("Name"="TestMode/TestName") -> ("String"=w204:string)  [unwired: 9 in, 1 out]
            n113 = call <vilib>:"NT Read and Format Entries as Tree.vi"("Operation"=w209, "Name Pattern"=w214, "Tree Refnum"=w215) -> ()  [unwired: 7 in, 2 out]
            n114 = case shown="\"\"" w204 {
              tunnel: "TestMode/TestProgress" ("Name") -> [w217 _]
              tunnel: "TestMode/TestProgressText" ("Name") -> [w216 _]
              frame Default {
                n115 = call <vilib>:"NT Read Number.vi"("Name"=w217) -> ("Numeric"=w218:dbl)  [unwired: 9 in, 1 out]
                n116 = call <vilib>:"NT Read String.vi"("Name"=w216) -> ("String"=w219:string)  [unwired: 9 in, 1 out]
                n117 = Bundle("Numeric"=w218, "String"=w219) -> (→"Progress":cluster{"Numeric":dbl, "String":string})  [unwired: 1 in]
              }
              frame "" {
                n118 = property on="Progress" class="Clust (strict)"("Visible"=FALSE) -> ()  [unwired: 2 in, 2 out]
                n119 = local write "Test Name"(u16 0) -> ()
              }
            }
            n120 = property on="Test Tree" class="Tree (strict)"("Active Item Row Number"=w213, "ActiveColNum"=w213, "CellBG"=w210, "Active Item Row Number"=-1 ("Active Item:Row Number"), "CellBG"=u32 5789784 ("Color Box")) -> ()  [unwired: 2 in, 2 out]
          }
          frame "Variables" {
            w225 = string[] ["CameraPublisher", "Usage", "DB"]  # Items to initially close
            n121 = First Call?() -> (First Call?: T/F=w226:bool)
            n122 = control-ref of="Tree"() -> (w227:refnum<vi>)
            n123 = Select(t=w225, s=w226, f=string[] []) -> (s? t:f=w223:string[])
            n124 = call <vilib>:"NT Read and Format Entries as Tree.vi"("Tags to  Close"=w223, "Tree Refnum"=w227) -> ()  [unwired: 8 in, 2 out]
          }
          frame "Commands" {
            w236 = u32 5789784 ("Color Box")
            w237 = T25 {"Row"=-1, "Column"=-2} ("Active Cell:Active Cell")
            w239 = T25 {"Row"=-2, "Column"=-2} ("Active Cell:Active Cell")
            n125 = Index Array(array=w240, index=w234) -> (element=w238:u32)
            n126 = Index Array(array=w235, index=w234) -> (element=w233:T24)
            n127 = Unbundle(w233) -> ("Operation"=w232:enum16{"Update", "Clear"})  [unwired: 1 out]
            n128 = local read "Command Selection"() -> (w231:i32)
            n129 = property on="Command Selection" class="MCListbox (strict)"("ActiveCell"=w239, "CellBG"=w238, "ActiveCell"=w237, "CellBG"=w236) -> ()  [unwired: 2 in, 2 out]
            n130 = call <vilib>:"WPI_DashboardUpdate RPC Info.vi"("Operation"=w232) -> ("update"=w230:bool, "commands"=w229:string[][])  [unwired: 9 in]
            n131 = property on="Command Selection" class="MCListbox (strict)"("ItemNames"=w229) -> ()  [unwired: 2 in, 2 out]
            n132 = property on="Command Params" class="Tbl (strict)"("Active Cell"=w239, "Cell BG Color"=w238, "Active Cell"=w237, "Cell BG Color"=w236) -> ()  [unwired: 2 in, 2 out]
            n133 = call <vilib>:"WPI_DashboardUpdate Command Params.vi"("Update"=w230, "NewVal"=w231, "Commands"=w229, "Param Tbl"=w228) -> ()  [unwired: 7 in, 1 out]
          }
        }
        n134 = call <vilib>:"Connextion Info.vi"() -> ("Connected"=→"NT Connection":bool)  [unwired: 10 in, 1 out]
      }
      event "Test Tree": Value Change {
        # "Show appropriate\ncontrols"
        n135 = event-data() -> ("CtlRef"=w245:refnum<vi>, "NewVal"=w243:string)  [unwired: 1 in]
        n136 = call <vilib>:"WPI_UtilitiesGetTreeIOName.vi"("NewVal"=w243, "TreeControl in"=w245) -> ("I/O Name"=w246:string)  [unwired: 9 in]
        n137 = case shown="\"Camera\"" w246 {
          selector: w246 -> [_ w253 _ w275 w284 _]
          tunnel: w243 -> [_ _ w272 w274 _ w291]
          tunnel: cluster{string[]}[] [{["640x480", "320x240", "160x120"]}, {["Auto", "Fixed indoor", "Fixed outdoor 1", "Fixed outdoor 2", "Fixed fluorescent 1", "Fixed fluorescent 2", "Hold current"]}, {["Auto", "Flicker-free 50 Hz", "Flicker-free 60 Hz", "Hold current"]}, {["None", "Prioritize frame rate", "Prioritize image quality"]}, {["Monochrome", "Color"]}] -> [_ _ _ _ _ w290]
          frame Default {
            w248 = FALSE ("Visible")
            w247 = FALSE ("Visible")
            n138 = property on="Motor" class="Clust (strict)"("Visible"=w247) -> ()  [unwired: 2 in, 2 out]
            n139 = property on="Test Ring" class="Ring (strict)"("Visible"=w247) -> ()  [unwired: 2 in, 2 out]
            n140 = property on="Rev/Fwd" class="Clust (strict)"("Visible"=w248) -> ()  [unwired: 2 in, 2 out]
            n141 = property on="On/Off" class="Bool (strict)"("Visible"=w248) -> ()  [unwired: 2 in, 2 out]
            n142 = property on="Test Slider" class="Slide (strict)"("Visible"=w248) -> ()  [unwired: 2 in, 2 out]
          }
          frame "Analog Out", "Motor", "PWM" {
            w254 = FALSE ("Visible")
            n143 = case shown="\"Analog Out\"" w253 {
              tunnel: [1.0 ("Value") -1.0 ("Value") 0.0 ("Value")] -> w252
              tunnel: [255.0 ("Value") 1.0 ("Value") 5.0 ("Value")] -> w251
              tunnel: [128.0 ("Value") 0.0 ("Value") 0.0 ("Value")] -> w250
              tunnel: [64.0 ("Value") 0.5 ("Value") 1.0 ("Value")] -> w249
              frame "PWM" {
              }
              frame "Motor", Default {
              }
              frame "Analog Out" {
              }
            }
            n144 = property on="Motor" class="Clust (strict)"("Visible"=TRUE) -> ()  [unwired: 2 in, 2 out]
            n145 = property on="Value" class="Slide (strict)"("Value"=w250, "Scale.Minimum"=w252, "Scale.Maximum"=w251, "Scale.Increment"=w249) -> ()  [unwired: 2 in, 2 out]
            n146 = property on="On/Off" class="Bool (strict)"("Visible"=w254) -> ()  [unwired: 2 in, 2 out]
            n147 = property on="Test Slider" class="Slide (strict)"("Visible"=w254) -> ()  [unwired: 2 in, 2 out]
            n148 = property on="Test Ring" class="Ring (strict)"("Visible"=w254) -> ()  [unwired: 2 in, 2 out]
            n149 = property on="Rev/Fwd" class="Clust (strict)"("Visible"=w254) -> ()  [unwired: 2 in, 2 out]
          }
          frame "Servo" {
            w270 = FALSE ("Visible")
            n150 = call <vilib>:"NT Read Number.vi"("Name"=w272) -> ("Numeric"=w271:dbl)  [unwired: 9 in, 1 out]
            n151 = property on="Test Slider" class="Slide (strict)"("Visible"=TRUE, "Scale.Maximum"=170.0 ("Scale.Range:Maximum")) -> ()  [unwired: 2 in, 2 out]
            n152 = local write "Test Slider"(w271) -> ()
            n153 = property on="Motor" class="Clust (strict)"("Visible"=w270) -> ()  [unwired: 2 in, 2 out]
            n154 = property on="Rev/Fwd" class="Clust (strict)"("Visible"=w270) -> ()  [unwired: 2 in, 2 out]
            n155 = property on="On/Off" class="Bool (strict)"("Visible"=w270) -> ()  [unwired: 2 in, 2 out]
            n156 = property on="Test Ring" class="Ring (strict)"("Visible"=w270) -> ()  [unwired: 2 in, 2 out]
          }
          frame "Relay", "Solenoid" {
            w273 = FALSE ("Visible")
            n157 = property on="Motor" class="Clust (strict)"("Visible"=w273) -> ()  [unwired: 2 in, 2 out]
            n158 = property on="Test Slider" class="Slide (strict)"("Visible"=w273) -> ()  [unwired: 2 in, 2 out]
            n159 = Search and Replace String(input string=w274, search string="/Value  **", replace string="/Direction") -> (result string=w280:string)  [unwired: 5 in, 3 out]
            n160 = property on="Test Ring" class="Ring (strict)"("Visible"=w273) -> ()  [unwired: 2 in, 2 out]
            n161 = call <vilib>:"NT Read String.vi"("Name"=w280) -> ("String"=w278:string)  [unwired: 9 in, 1 out]
            n162 = Equal?(x="Both directions", y=w278) -> (x = y?=w276:bool)
            n163 = Not(x=w276) -> (.not. x?=w277:bool)
            n164 = property on="Rev/Fwd" class="Clust (strict)"("Visible"=w276) -> ()  [unwired: 2 in, 2 out]
            n165 = property on="On/Off" class="Bool (strict)"("Visible"=w277, "Caption.Text"=w275) -> ()  [unwired: 2 in, 2 out]
          }
          frame "Compressor", "Digital Out" {
            w283 = FALSE ("Visible")
            # "Get direction and finish"
            n166 = property on="Motor" class="Clust (strict)"("Visible"=w283) -> ()  [unwired: 2 in, 2 out]
            n167 = property on="Test Slider" class="Slide (strict)"("Visible"=w283) -> ()  [unwired: 2 in, 2 out]
            n168 = property on="Test Ring" class="Ring (strict)"("Visible"=w283) -> ()  [unwired: 2 in, 2 out]
            n169 = property on="On/Off" class="Bool (strict)"("Visible"=TRUE, "Caption.Text"=w284) -> ()  [unwired: 2 in, 2 out]
            n170 = property on="Rev/Fwd" class="Clust (strict)"("Visible"=FALSE) -> ()  [unwired: 2 in, 2 out]
          }
          frame "Camera" {
            n171 = call <vilib>:"Get Last Path Segment.vi"("String in"=w291) -> ("String out"=w292:string)  [unwired: 10 in]
            n172 = property on="On/Off" class="Bool (strict)"("Visible"=FALSE) -> ()  [unwired: 2 in, 2 out]
            n173 = property on="Motor" class="Clust (strict)"("Visible"=FALSE) -> ()  [unwired: 2 in, 2 out]
            n174 = property on="Rev/Fwd" class="Clust (strict)"("Visible"=FALSE) -> ()  [unwired: 2 in, 2 out]
            n175 = case shown="\"White Balance  **\"" w292 {
              tunnel: w291 -> [w298 w307 w316 w325 w334 _ w340]
              tunnel: w290 -> [w296 w304 w313 w322 w331 _ _]
              frame "Size  **" {
                n176 = Index Array(array=w296) -> (element=w295:cluster{string[]})  [unwired: 1 in]
                n177 = call <vilib>:"NT Read String.vi"("Name"=w298) -> ("String"=w297:string)  [unwired: 9 in, 1 out]
                n178 = Unbundle(w295) -> (w293:string[])
                n179 = Match First String(2:w293, 3:w297) -> (0:w294:i32)  [unwired: 1 out]
                n180 = property on="Test Ring" class="Ring (strict)"("Value"=w294, "Strings []"=w293) -> ()  [unwired: 2 in, 2 out]
                n181 = property on="Test Ring" class="Ring (strict)"("Visible"=TRUE) -> ()  [unwired: 2 in, 2 out]
                n182 = property on="Test Slider" class="Slide (strict)"("Visible"=FALSE) -> ()  [unwired: 2 in, 2 out]
              }
              frame "White Balance  **" {
                n183 = Index Array(array=w304, index=1) -> (element=w305:cluster{string[]})
                n184 = call <vilib>:"NT Read String.vi"("Name"=w307) -> ("String"=w306:string)  [unwired: 9 in, 1 out]
                n185 = Unbundle(w305) -> (w302:string[])
                n186 = Match First String(2:w302, 3:w306) -> (0:w301:i32)  [unwired: 1 out]
                n187 = property on="Test Ring" class="Ring (strict)"("Value"=w301, "Strings []"=w302) -> ()  [unwired: 2 in, 2 out]
                n188 = property on="Test Ring" class="Ring (strict)"("Visible"=TRUE) -> ()  [unwired: 2 in, 2 out]
                n189 = property on="Test Slider" class="Slide (strict)"("Visible"=FALSE) -> ()  [unwired: 2 in, 2 out]
              }
              frame "Exposure  **" {
                n190 = Index Array(array=w313, index=2) -> (element=w314:cluster{string[]})
                n191 = call <vilib>:"NT Read String.vi"("Name"=w316) -> ("String"=w315:string)  [unwired: 9 in, 1 out]
                n192 = Unbundle(w314) -> (w310:string[])
                n193 = Match First String(2:w310, 3:w315) -> (0:w311:i32)  [unwired: 1 out]
                n194 = property on="Test Ring" class="Ring (strict)"("Value"=w311, "Strings []"=w310) -> ()  [unwired: 2 in, 2 out]
                n195 = property on="Test Ring" class="Ring (strict)"("Visible"=TRUE) -> ()  [unwired: 2 in, 2 out]
                n196 = property on="Test Slider" class="Slide (strict)"("Visible"=FALSE) -> ()  [unwired: 2 in, 2 out]
              }
              frame "Exposure Priority  **" {
                n197 = Index Array(array=w322, index=3) -> (element=w323:cluster{string[]})
                n198 = call <vilib>:"NT Read String.vi"("Name"=w325) -> ("String"=w324:string)  [unwired: 9 in, 1 out]
                n199 = Unbundle(w323) -> (w319:string[])
                n200 = Match First String(2:w319, 3:w324) -> (0:w320:i32)  [unwired: 1 out]
                n201 = property on="Test Ring" class="Ring (strict)"("Value"=w320, "Strings []"=w319) -> ()  [unwired: 2 in, 2 out]
                n202 = property on="Test Ring" class="Ring (strict)"("Visible"=TRUE) -> ()  [unwired: 2 in, 2 out]
                n203 = property on="Test Slider" class="Slide (strict)"("Visible"=FALSE) -> ()  [unwired: 2 in, 2 out]
              }
              frame "Color Enable  **" {
                n204 = Index Array(array=w331, index=4) -> (element=w332:cluster{string[]})
                n205 = call <vilib>:"NT Read String.vi"("Name"=w334) -> ("String"=w333:string)  [unwired: 9 in, 1 out]
                n206 = Unbundle(w332) -> (w328:string[])
                n207 = Match First String(2:w328, 3:w333) -> (0:w329:i32)  [unwired: 1 out]
                n208 = property on="Test Ring" class="Ring (strict)"("Value"=w329, "Strings []"=w328) -> ()  [unwired: 2 in, 2 out]
                n209 = property on="Test Ring" class="Ring (strict)"("Visible"=TRUE) -> ()  [unwired: 2 in, 2 out]
                n210 = property on="Test Slider" class="Slide (strict)"("Visible"=FALSE) -> ()  [unwired: 2 in, 2 out]
              }
              frame Default {
                n211 = property on="Test Ring" class="Ring (strict)"("Visible"=FALSE) -> ()  [unwired: 2 in, 2 out]
                n212 = property on="Test Slider" class="Slide (strict)"("Visible"=FALSE) -> ()  [unwired: 2 in, 2 out]
              }
              frame "Brightness  **", "Color Level  **", "Compression  **", "FPS  **", "Sharpness  **" {
                n213 = call <vilib>:"NT Read Number.vi"("Name"=w340) -> ("Numeric"=w339:dbl)  [unwired: 9 in, 1 out]
                n214 = local write "Test Slider"(w339) -> ()
                n215 = property on="Test Slider" class="Slide (strict)"("Visible"=TRUE, "Scale.Maximum"=100.0 ("Scale.Range:Maximum")) -> ()  [unwired: 2 in, 2 out]
                n216 = property on="Test Ring" class="Ring (strict)"("Visible"=FALSE) -> ()  [unwired: 2 in, 2 out]
              }
            }
          }
        }
        n217 = property on="Progress" class="Clust (strict)"("Visible"=FALSE) -> ()  [unwired: 2 in, 2 out]
      }
      event "Test Name": Mouse Enter {
        # "Populate the ring with the list of tests"
        n218 = event-data() -> ()  [unwired: 1 in, 1 out]
        n219 = call <vilib>:"NT Read String Array.vi"("Name"="TestMode/TestList") -> ("String Array"=w348:string[])  [unwired: 9 in, 1 out]
        n220 = Build Array (concatenate)("Select the test to run...", w348) -> (w347:string[])
        n221 = property on="Test Name" class="Ring (strict)"("Strings []"=w347) -> ()  [unwired: 2 in, 2 out]
      }
      event "Test Name": Value Change {
        w350 = FALSE ("Visible")
        # "Tell the robot the test name to run"
        n222 = event-data() -> ("NewVal"=w354:u16)  [unwired: 1 in]
        n223 = property on="Test Name" class="Ring (strict)"() -> ("Strings []"=w355:string[])  [unwired: 2 in, 2 out]
        n224 = local write "Progress"(T6 {"Test Progress"=0, "Test Progress Text"=""} ("Progress")) -> ()
        n225 = Index Array(array=w355, index=w354) -> (element=w353:string)
        n226 = call <vilib>:"NT Write String.vi"("String"=w353, "Name"="TestMode/TestName") -> ()  [unwired: 9 in, 1 out]
        n227 = property on="Progress" class="Clust (strict)"("Visible"=TRUE) -> ()  [unwired: 2 in, 2 out]
        n228 = property on="Motor" class="Clust (strict)"("Visible"=w350) -> ()  [unwired: 2 in, 2 out]
        n229 = property on="Test Slider" class="Slide (strict)"("Visible"=w350) -> ()  [unwired: 2 in, 2 out]
        n230 = property on="On/Off" class="Bool (strict)"("Visible"=w350) -> ()  [unwired: 2 in, 2 out]
        n231 = property on="Rev/Fwd" class="Clust (strict)"("Visible"=w350) -> ()  [unwired: 2 in, 2 out]
        n232 = property on="Test Ring" class="Ring (strict)"("Visible"=w350) -> ()  [unwired: 2 in, 2 out]
      }
      event "Select Auto": Mouse Enter {
        # "Populate the combo box with the list of autonomous options"
        n233 = event-data() -> ()  [unwired: 1 in, 1 out]
        n234 = call <vilib>:"NT Read String Array.vi"("Name"="Auto List") -> ("String Array"=w357:string[])  [unwired: 9 in, 1 out]
        n235 = property on="Select Auto" class="CmbBox"("Strings[]"=w357) -> ()  [unwired: 2 in, 2 out]
      }
      event "Select Auto": Value Change {
        # "User modified the Auto Selection. Write to NT variable so robot knows."
        n236 = event-data() -> ("NewVal"=w360:string)  [unwired: 1 in]
        n237 = call <vilib>:"NT Write String.vi"("String"=w360, "Name"="Auto Selector") -> ()  [unwired: 9 in, 1 out]
      }
      event "Command Selection": Value Change {
        # "Get the params and show in table"
        n238 = event-data() -> ("NewVal"=w366:i32)  [unwired: 1 in]
        n239 = property on="Command Selection" class="MCListbox (strict)"() -> ("ItemNames"=w364:string[][])  [unwired: 2 in, 2 out]
        n240 = call <vilib>:"WPI_DashboardUpdate Command Params.vi"("NewVal"=w366, "Commands"=w364, "Param Tbl"=w365) -> ()  [unwired: 8 in, 1 out]
      }
      event "Execute Command": Value Change {
        # "Started one, Unique ID holds\nresponse"
        n241 = event-data() -> ()  [unwired: 1 in, 1 out]
        n242 = property on="Command Selection" class="MCListbox (strict)"() -> ("ItemNames"=w377:string[][])  [unwired: 2 in, 2 out]
        n243 = Index Array(array=w377, index (row)="Command Selection", index (col)=0) -> (element=w375:string)
        n244 = call <vilib>:"Invoke Commands.vi"("Command Params"="Command Params", "Function Name"=w375) -> ("Params"=w371:u8, "Started"=w370:bool)  [unwired: 7 in, 1 out]
        n245 = Array Subset(array="Command Params", length (row)=w371) -> (w372:string[][])  [unwired: 3 in]
        n246 = Select(t="Executing" ("Cmd Status"), s=w370, f="" ("Cmd Status")) -> (s? t:f=→"Cmd Status":string)
      }
      event "Command Selection": Double Click {
        n247 = event-data() -> ("Row"=w385:i32)  [unwired: 1 in]
        n248 = property on="Command Selection" class="MCListbox (strict)"() -> ("ItemNames"=w388:string[][])  [unwired: 2 in, 2 out]
        n249 = local read "Command Params"() -> (w384:string[][])
        n250 = Index Array(array=w388, index (row)=w385, index (col)=0) -> (element=w386:string)
        n251 = call <vilib>:"Invoke Commands.vi"("Command Params"=w384, "Function Name"=w386) -> ("Params"=w383:u8, "Started"=w378:bool)  [unwired: 7 in, 1 out]
        n252 = Array Subset(array=w384, length (row)=w383) -> (w382:string[][])  [unwired: 3 in]
        n253 = Select(t="Executing" ("Cmd Status"), s=w378, f="" ("Cmd Status")) -> (s? t:f=w379:string)
        n254 = local write "Cmd Status"(w379) -> ()
      }
      event "CheckList": Double Click {
        # "Shift clears all"
        # "Update symbols on the listbox"
        n255 = event-data() -> ("PlatMods.Shift"=w390:bool, "Row"=w392:i32)  [unwired: 1 in]
        n256 = case shown="True" w390 {
          tunnel: w392 -> [w396 _]
          tunnel: 1 -> [w395 _]
          frame False {
            n257 = property on="CheckList" class="LstBox (strict)"() -> ("Item Symbols"=w394:i32[])  [unwired: 2 in, 2 out]
            n258 = Replace Array Subset(array=w394, new element=w395, index=w396) -> (w393:i32[])
            n259 = property on="CheckList" class="LstBox (strict)"("Item Symbols"=w393) -> ()  [unwired: 2 in, 2 out]
          }
          frame True {
            w397 = 0 ("Top Row")
            n260 = property on="CheckList" class="LstBox (strict)"() -> ("Number of Rows"=w399:u32)  [unwired: 2 in, 2 out]
            n261 = Initialize Array(0, w399) -> (w398:i32[])
            n262 = property on="CheckList" class="LstBox (strict)"("Top Row"=w397, "Value"=w397, "Item Symbols"=w398) -> ()  [unwired: 2 in, 2 out]
          }
        }
      }
      event "CheckList": Key Down {
        # "Update symbols on the listbox\nLeft and right keys check and uncheck"
        n263 = event-data() -> ("VKey"=w403:T22)  [unwired: 1 in]
        n264 = case shown="\"Left\", \"Right\"" w403 {
          selector: w403 -> [w408 _]
          tunnel: eventvkey."Left" ("VKey") -> [w406 _]
          frame "Left", "Right" {
            n265 = Equal?(x=w406, y=w408) -> (x = y?=w407:bool)
            n266 = Select(t=0, s=w407, f=1) -> (s? t:f=w409:i32)
            n267 = property on="CheckList" class="LstBox (strict)"() -> ("Item Symbols"=w412:i32[])  [unwired: 2 in, 2 out]
            n268 = Replace Array Subset(array=w412, new element=w409, index="CheckList") -> (w411:i32[])
            n269 = property on="CheckList" class="LstBox (strict)"("Item Symbols"=w411) -> ()  [unwired: 2 in, 2 out]
          }
          frame Default {
          }
        }
      }
      event "Motor.Enable": Value Change {
        # "When the test mode otor enable helper is set, update that\ntree row item's value"
        n270 = event-data() -> ("NewVal"=w418:bool)  [unwired: 1 in]
        n271 = Unbundle("Motor") -> ("Value"=w417:dbl)  [unwired: 1 out]
        n272 = Select(t=w417, s=w418, f=0.0) -> (s? t:f=w415:dbl)
        n273 = call <vilib>:"NT Write Number.vi"("Numeric"=w415, "Name"=w414) -> ()  [unwired: 9 in, 1 out]
      }
      event "Test Slider": Value Change {
        # "When the test mode slider helper is set, update that\ntree row item's value"
        n274 = event-data() -> ("NewVal"=w421:dbl)  [unwired: 1 in]
        n275 = call <vilib>:"NT Write Number.vi"("Numeric"=w421, "Name"=w422) -> ()  [unwired: 9 in, 1 out]
      }
      event "On/Off": Value Change {
        # "When the test mode on/off helper value is set, update that\ntree row item's value"
        n276 = event-data() -> ("NewVal"=w426:bool)  [unwired: 1 in]
        n277 = Boolean To (0,1)(Boolean=w426) -> (0, 1=w425:i16)
        n278 = call <vilib>:"NT Write Number.vi"("Numeric"=w425, "Name"=w424) -> ()  [unwired: 9 in, 1 out]
      }
      event "Rev/Fwd": Value Change {
        # "When the test mode helper value for relays is set, update that\ntree row item's value"
        n279 = event-data() -> ("NewVal.Forward"=w434:bool, "NewVal.Reverse"=w433:bool)  [unwired: 1 in]
        n280 = Boolean To (0,1)(Boolean=w434) -> (0, 1=w430:i16)
        n281 = Boolean To (0,1)(Boolean=w433) -> (0, 1=w432:i16)
        n282 = Negate(x=w432) -> (-x=w431:i16)
        n283 = Add(x=w430, y=w431) -> (x+y=w429:i16)
        n284 = call <vilib>:"NT Write Number.vi"("Numeric"=w429, "Name"=w428) -> ()  [unwired: 9 in, 1 out]
      }
      event "Test Ring": Value Change {
        # "When a test mode helper value is selected from the ring,\nset the tree item's variable to the string value"
        n285 = event-data() -> ("NewVal"=w438:u16)  [unwired: 1 in]
        n286 = property on="Test Ring" class="Ring (strict)"() -> ("Strings []"=w439:string[])  [unwired: 2 in, 2 out]
        n287 = Index Array(array=w439, index=w438) -> (element=w437:string)
        n288 = call <vilib>:"NT Write String.vi"("String"=w437, "Name"=w436) -> ()  [unwired: 9 in, 1 out]
      }
      event "Rec Mode": Value Change {
        # "Update globals for recording mode and path to read log from.\nClear when logging and let NetworkTables set path for vision to\nuse."
        n289 = event-data() -> ("NewVal"=w450:enum32{"Stop", "Record", "Playback"})  [unwired: 1 in]
        n290 = global write "WPI_DashboardLogging Global.vi" "Logging Filename"(path "") -> ()
        n291 = global write "WPI_DashboardLogging Global.vi" "Recording"(w450) -> ()
        n292 = case shown="\"Playback\"" w450 {
          tunnel: w449 -> [_ w452 w461]
          tunnel: [_ _ w460] -> w447
          tunnel: [_ _ w459] -> _
          tunnel: w445 -> [_ _ w457]
          tunnel: cluster{i32, i32} {-250, 170} -> [_ _ w456]
          tunnel: [_ _ T23 {"Image Size"=TRUE, "Image Type"=TRUE, "Pixel Value"=TRUE, "ROI Information"=TRUE, "Zoom Factor"=FALSE} ("Image Information Shown:All Elements")] -> w440
          tunnel: [_ _ TRUE ("Zoom Factor")] -> w441
          tunnel: w443 -> [_ _ w453]
          frame Default {
          }
          frame "Stop", "Record" {
            # "Place Window too"
            n293 = invoke class="VI" method="FP.Close"(reference=w452) -> (reference out=w451:refnum<vi>)  [unwired: 2 in, 2 out]
            n294 = invoke class="VI" method="Abort VI"(reference=w451) -> ()  [unwired: 2 in, 3 out]
          }
          frame "Playback" {
            n295 = call "Open Playback Panel.vi"("Offset"=w456, "DB VI Ref"=w457, "Playback in"=w461) -> ("Playback out"=w458:refnum<vi>)  [unwired: 8 in]
            n296 = register-events(w458, w453) -> (reference out=w460:refnum<event-registration>, error out=w459:errorcluster)  [unwired: 2 in]
          }
        }
        n297 = property on="Camera Image Right" class="ImageControl"("Image Information Shown"=w440, "Image Information Visible"=w441) -> ()  [unwired: 2 in, 2 out]
        n298 = property on="Camera Image" class="ImageControl"("Image Information Shown"=w440, "Image Information Visible"=w441) -> ()  [unwired: 2 in, 2 out]
        n299 = call <vilib>:"WPI_DashboardNT Log FieldName Cache.vi"("Operation"=enum16{"Lookup/Add", "Index", "Clear"}."Clear") -> ()  [unwired: 8 in, 3 out]
      }
      event Panel Close {
        w463 = enum32{"Stop", "Record", "Playback"}."Stop" ("Rec Mode")
        # "Playback window has been closed, abort"
        n300 = event-data() -> ()  [unwired: 1 in, 4 out]
        n301 = local write "Rec Mode"(w463) -> ()
        n302 = global write "WPI_DashboardLogging Global.vi" "Recording"(w463) -> ()
      }
      event Panel Close {
        # "Abort playback window and ourself"
        n303 = event-data() -> ()  [unwired: 1 in, 4 out]
        n304 = invoke class="VI" method="FP.Close"(reference=w467) -> (reference out=w466:refnum<vi>)  [unwired: 2 in, 2 out]
        n305 = invoke class="VI" method="Abort VI"(reference=w466) -> (error out=w465:errorcluster)  [unwired: 2 in, 2 out]
        n306 = invoke class="VI" method="Abort VI"(error in=w465) -> ()  [unwired: 2 in, 3 out]
      }
      event User Event {
        n307 = event-data() -> ("IDs"=w474:cluster{"RPC field ID":u16, "Unique ID":u16}, "String"=w473:string)  [unwired: 1 in]
        n308 = Bundle("IDs"=w474, "String"=w473) -> (w472:T9)  [unwired: 1 in]
        n309 = call <vilib>:"Retrieve RPC Response.vi"("RPC Response"=w472) -> ("Output"=w470:string[][])  [unwired: 10 in]
        n310 = Build Array (concatenate)(w468, w470) -> (w469:string[][])
        n311 = local write "Command Params"(w469) -> ()
        n312 = local write "Cmd Status"("" ("Cmd Status")) -> ()
      }
      event "Tree": Double Click {
        n313 = event-data() -> ("PlatMods"=w480:T26, "Tag"=w477:string)  [unwired: 1 in]
        n314 = Unbundle(w480) -> ("Shift"=w479:bool)  [unwired: 4 out]
        n315 = String Subset(string=w477, length (rest)=1 ("length (rest)")) -> (substring=w476:string)  [unwired: 1 in]
        n316 = Not(x=w479) -> (.not. x?=w478:bool)
        n317 = case shown="\"/\"" w476 {
          tunnel: w477 -> [_ w483]
          tunnel: w478 -> [_ w482]
          frame Default {
          }
          frame "/" {
            n318 = call <vilib>:"NT Update Persistence.vi"("Persistence"=w482, "Name"=w483) -> ()  [unwired: 9 in, 1 out]
          }
        }
      }
    }
  }
  n319 = while {
    tunnel: w65 -> [w485]
    i -> [w488]
    stop <- FALSE stop-if-true
    n320 = Wait (ms)(milliseconds to wait=u32 100) -> ()  [unwired: 1 out]
    n321 = case shown="\"Playback\"" "Rec Mode" {
      tunnel: w488 -> [_ _ w503]
      tunnel: [u32 2829099 ("Base Color") u32 11141120 ("Target Color") w492] -> w484
      frame "Stop", Default {
        # "Reset the color, extra updates don't cost much"
      }
      frame "Record" {
      }
      frame "Playback" {
        # "Playback"
        n322 = Quotient & Remainder(x=w503, y=u32 50 ("milliseconds to wait")) -> (x-y*floor(x/y)=w499:u32)  [unwired: 1 out]
        n323 = Divide(x=w499, y=u32 50 ("milliseconds to wait")) -> (x/y=w496:dbl)
        n324 = Multiply(x=6.283185307179586, y=w496) -> (x*y=w501:dbl)
        n325 = Sine(x=w501) -> (sin(x)=w500:dbl)
        n326 = Absolute Value(x=w500) -> (abs(x)=w493:dbl)
        n327 = call "Interpolate RGB Color.vi"("Proportion"=w493, "Target Color"=u32 30976, "Base Color"=u32 2829099) -> ("Result Color"=w492:u32)  [unwired: 8 in]
      }
    }
    n328 = property class="Pane"(reference=w485, "PaneColor"=w484) -> ()  [unwired: 1 in, 2 out]
  }
  n329 = local write "Dashboard Tab"(T2."Drive" ("Dashboard Tab")) -> ()
  n330 = property on="On/Off" class="Bool (strict)"("Visible"=w36) -> ()  [unwired: 2 in, 2 out]
  n331 = property on="Motor" class="Clust (strict)"("Visible"=w36) -> ()  [unwired: 2 in, 2 out]
  n332 = property on="Progress" class="Clust (strict)"("Visible"=w36) -> ()  [unwired: 2 in, 2 out]
  n333 = property on="Test Ring" class="Ring (strict)"("Visible"=w36) -> ()  [unwired: 2 in, 2 out]
  n334 = property on="Rev/Fwd" class="Clust (strict)"("Visible"=w36) -> ()  [unwired: 2 in, 2 out]
  n335 = while {
    tunnel: u16 1741 ("timeout ms (25000)") -> [w505]
    stop <- FALSE stop-if-true
    n336 = TCP Create Listener(10:w505) -> (0:w504:errorcluster, 3:w506:refnum<k5>)  [unwired: 4 in, 1 out]
    n337 = case shown="No Error" w504 {
      selector: w504 -> [w508 _]
      tunnel: w506 -> [w509 _]
      frame No Error {
        n338 = while {
          tunnel: w509 -> [w512]
          tunnel: w508 -> [w511]
          stop <- FALSE stop-if-true
          n339 = TCP Wait On Listener(8:w511, 11:w512) -> (0:w513:errorcluster, 4:w514:refnum<k5>)  [unwired: 2 in, 3 out]
          n340 = local write "TCP"(w514) -> ()
          n341 = case shown="No Error" w513 {
            frame No Error {
            }
            frame Error {
              n342 = Wait (ms)(milliseconds to wait=u32 1000) -> ()  [unwired: 1 out]
            }
          }
        }
      }
      frame Error {
        n343 = Wait (ms)(milliseconds to wait=u32 1000) -> ()  [unwired: 1 out]
      }
    }
  }
  n344 = local write "Command Selection"(u16 0 ("milliseconds to wait")) -> ()
  n345 = local write "Command Params"(string[][] [] ("Command Params")) -> ()
  n346 = global write "WPI_DashboardLogging Global.vi" "Recording"(w59) -> ()
  n347 = local write "Rec Mode"(w59) -> ()
  n348 = call <vilib>:"NT Write String.vi"("String"="Select Auto", "Name"="Auto Selector") -> ()  [unwired: 9 in, 1 out]
